vi "Prepend Array Element.vi"(8 "error in (no error)":errorcluster, 9 "JSON Value in":refnum<class "JSON Value.lvclass">, 11 "JSON Value in":refnum<class "JSON Value.lvclass">) -> (0 "error out":errorcluster, 2 "JSON Value out":refnum<class "JSON Value.lvclass">)   [LabVIEW 2016, in "JSON Value.lvclass"]
doc: "Prepends an array element to an existing JSON Array"
uses:
  JSON Value.lvclass
  JSON Value.lvclass/JSON Value.ctl
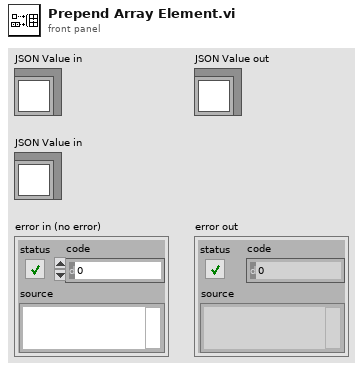
[diagram p1: front panel]
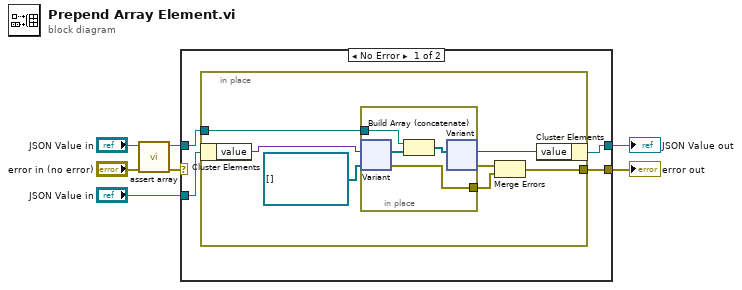
[diagram p0: block diagram]
diagram:
  n1 = call "assert array.vi"("error in (no error)"="error in (no error)", "JSON Value in"="JSON Value in") -> ("error out"=w3:errorcluster, "JSON Value out"=w1:refnum<class "JSON Value.lvclass">)  [unwired: 8 in]
  n2 = case shown="No Error" w3 {
    selector: w3 -> [_ w23]
    tunnel: "JSON Value in" -> [w11 _]
    tunnel: [w10 w24] -> w6
    tunnel: w1 -> [w9 w24]
    tunnel: [w8 w23] -> w5
    frame No Error {
      n3 = in-place {
        in-place-border: w9 -> [w18]
        in-place-border: [w12] -> w8
        n4 = in-place-cluster #1(w11) -> ("value"=w17:variant)
        n5 = in-place {
          in-place-border: w18 -> [w22]
          in-place-border: [w19] -> w13
          n6 = in-place-variant #2(w17, refnum<class "JSON Value.lvclass">[] [] ("JSON in")) -> (w21:refnum<class "JSON Value.lvclass">[], w19:errorcluster)
          n7 = Build Array (concatenate)(w22, w21) -> (w20:refnum<class "JSON Value.lvclass">[])
          n8 = in-place-variant #2(w20) -> (w15:variant, w14:errorcluster)
        }
        n9 = Merge Errors(w14, w13) -> (w12:errorcluster)
        n10 = in-place-cluster #1("value"=w15) -> (w10:refnum<class "JSON Value.lvclass">)
      }
    }
    frame Error {
    }
  }
  "JSON Value out" <- w6
  "error out" <- w5
